vi "Lockin.Remote Client.vi"(6 "timeout (ms) [20000]":i32=20000, 8 "error in (no error)":errorcluster, 9 "Data":variant, 10 "Command":variant, 11 "Instrument.Lockin in":refnum<class "Instrument.Lockin.lvclass">) -> (0 "error out":errorcluster, 1 "Data out":variant, 3 "Instrument.Lockin out":refnum<class "Instrument.Lockin.lvclass">)   [LabVIEW 2019, in "Instrument.Lockin.lvlib" / "Instrument.Lockin.lvclass"]
uses:
  Instrument.Lockin.lvclass
  C:/Program Files (x86)/National Instruments/LabVIEW 2019/user.lib/LevyLab/Instrument Framework/Instrument/Instrument.lvclass
  <userlib>/LevyLab/Instrument Framework/Instrument/Instrument.lvclass
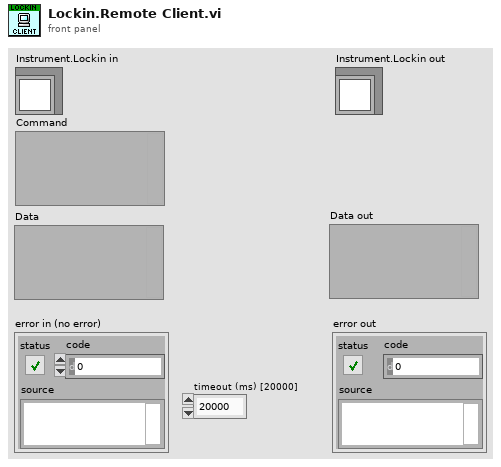
[diagram p1: front panel]
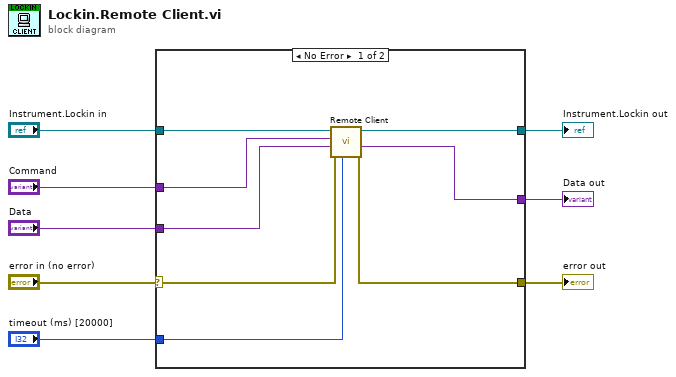
[diagram p0: block diagram]
diagram:
  n1 = case shown="No Error" "error in (no error)" {
    selector: "error in (no error)" -> [w12 w18]
    tunnel: "Data" -> [w16 _]
    tunnel: [w11 w18] -> w7
    tunnel: [w13 _] -> w6
    tunnel: "Command" -> [w9 _]
    tunnel: "Instrument.Lockin in" -> [w14 w17]
    tunnel: [w15 w17] -> w2
    tunnel: "timeout (ms) [20000]" -> [w10 _]
    frame No Error {
      n2 = call <userlib>:"Remote Client.vi"("timeout (ms) [500]"=w10, "error in (no error)"=w12, "Data in"=w16, "Command in"=w9, "Instrument in"=w14) -> ("error out"=w11:errorcluster, "Data out"=w13:variant, "Instrument out"=w15:refnum<class "Instrument.Lockin.lvclass">)  [unwired: 3 in, 1 out]
    }
    frame Error {
    }
  }
  "Instrument.Lockin out" <- w2
  "error out" <- w7
  "Data out" <- w6
